vi "Add State(s) to Queue By BOOL(Element).vi"(4 "False(\"\")":string, 6 "TRUE(\"\")":string, 8 "High Priority(FALSE)":bool, 10 "Bool":bool, 11 "State Queue(\"\")":string) -> (3 "State Queue Out":string)   [LabVIEW 2020, in "Communicable State Machine.lvlib"]
doc: "Depending on the High Priority and Bool input, this VI generates a concatenated state of TRUE/False and Remaining States. The High Priority input determines if the TRUE or False string concatenates before/after the remaining states. The Bool input determines whether TRUE or False string to be concatenated.\n\n<b>Inputs:</b>\n - <b>State Queue(\"\")</b>: The entire state queue is wired to this input.\n - <b>TRUE(\"\")</b>: State to insert when <b>Bool</b> is True.\n - <b>False(\"\")</b>: State to insert when <b>Bool</b> is False.\n - <b>Bool</b>: Flag for choosing State String connected to TRUE terminal or False terminal.\n - <b>High Priority(FALSE)</b>: If True, The state will be inserted to the top of the <b>State Queue(\"\")</b>. If False, It's appended to the tail.\n\n<b>Outputs:</b>\n - <b>State Queue Out</b>: Returns all the next states that should execute after the current state completes."
uses:
  Communicable State Machine.lvlib
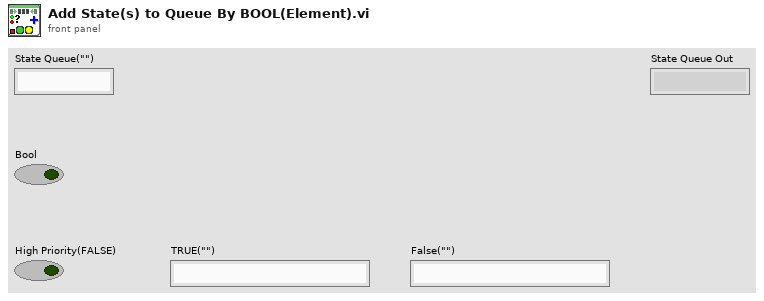
[diagram p1: front panel]
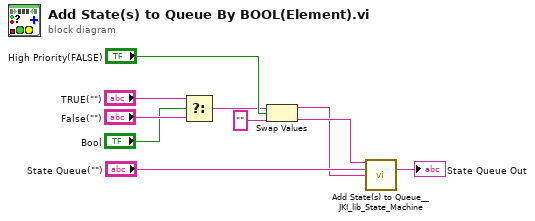
[diagram p0: block diagram]
diagram:
  n1 = Select(t="TRUE(\"\")", s="Bool", f="False(\"\")") -> (s? t:f=w4:string)
  n2 = Swap Values(12:w4, 13:"High Priority(FALSE)", 14:"") -> (1:w1:string, 3:w2:string)
  n3 = call "Add State(s) to Queue__JKI_lib_State_Machine.vi"("State(s) in Front (\"\")"=w2, "State(s) in (\"\")"="State Queue(\"\")", "State(s) at Back (\"\")"=w1) -> ("States Out"=→"State Queue Out":string)  [unwired: 12 in]
